vi "Attitude Control Write.vi"(8 "error in (no error)":errorcluster, 9 "Attitude in radians":cluster{"Roll":dbl, "Pitch":dbl, "Yaw":dbl}, 11 "Attitude Control Handle In":T1) -> (0 "error out":errorcluster, 3 "Attitude Control Handle Out":T1)   [LabVIEW 2013, in "lv-attitudecontrol.lvlib"]
uses:
  lv-attitudecontrol.lvlib
  Controls/AttitudeHandle.ctl
  <vilib>/Utility/miscctls.llb/LV3DPointTypeDef.ctl
  <vilib>/picture/3D Picture Control/NI_3D Picture Control.lvlib
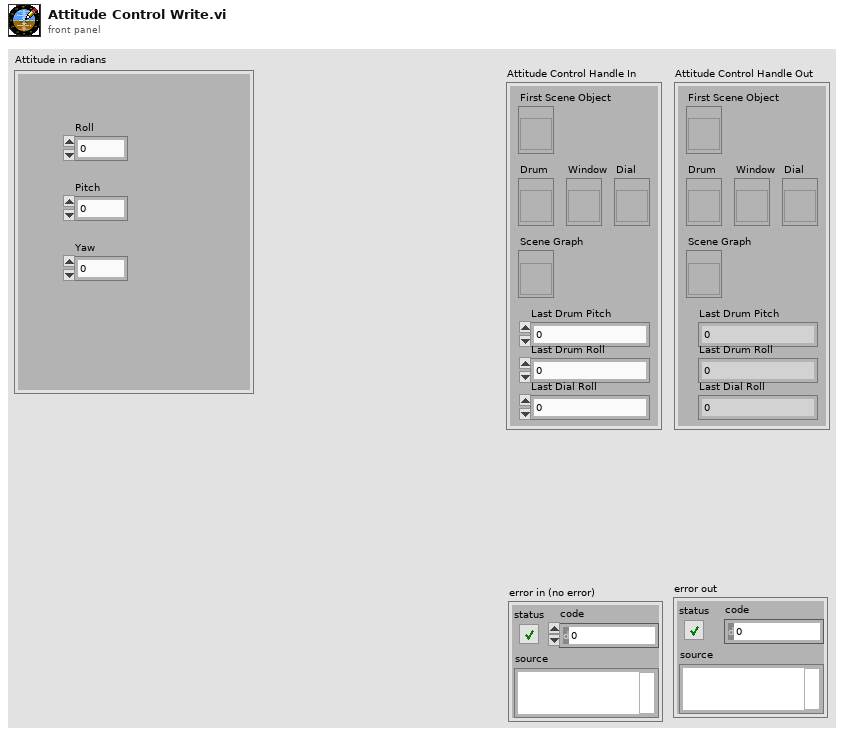
[diagram p1: front panel]
types:
  T1 = typedef "lv-attitudecontrol.lvlib/AttitudeHandle.ctl" = cluster{"First Scene Object":refnum<vi>, "Drum":refnum<vi>, "Window":refnum<vi>, "Dial":refnum<vi>, "Scene Graph":refnum<vi>, "Last Drum Pitch":dbl, "Last Drum Roll ":dbl, "Last Dial Roll":dbl}
  T2 = enum16{"None", "Spherical", "Flying", "Oriented"}
  T3 = typedef "LV3DPointTypeDef.ctl" = cluster{"X":sgl, "Y":sgl, "Z":sgl}
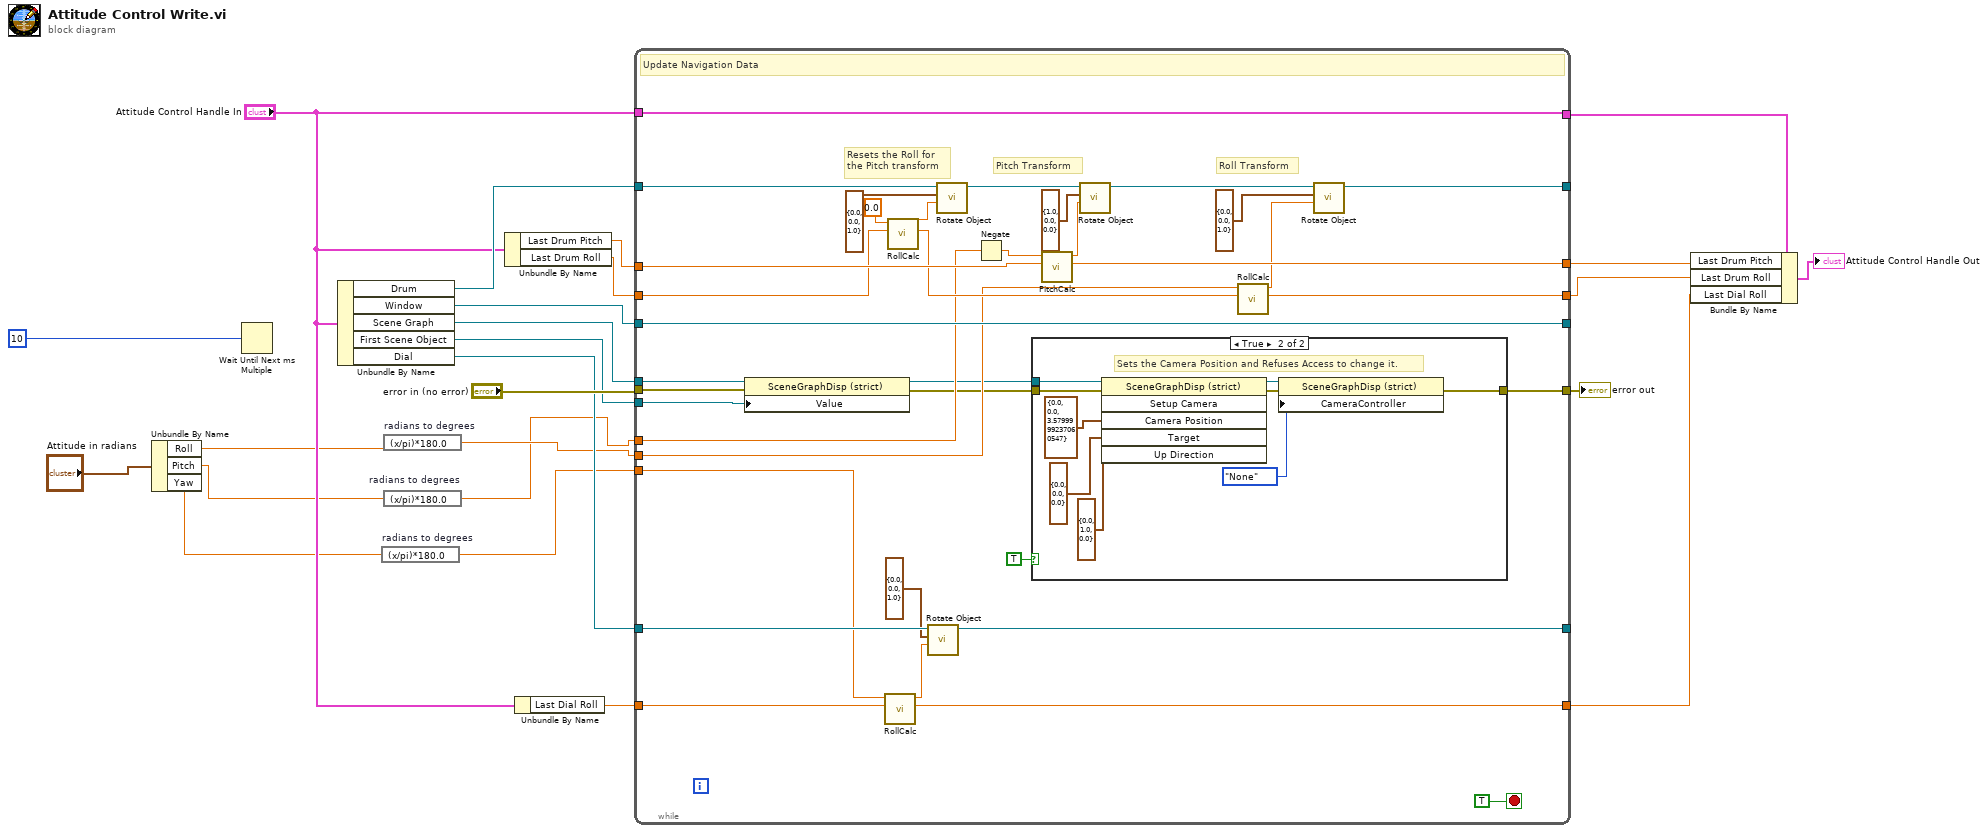
[diagram p0: block diagram]
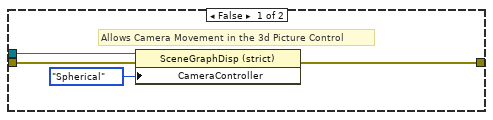
[diagram p2: hidden frame]
diagram:
  n1 = Unbundle By Name("Attitude in radians") -> ("Roll"=w7:dbl, "Pitch"=w6:dbl, "Yaw"=w5:dbl)
  n2 = Wait Until Next ms Multiple(millisecond multiple=u32 10) -> ()  [unwired: 1 out]
  n3 = Unbundle By Name("Attitude Control Handle In") -> ("Drum"=w22:refnum<vi>, "Window"=w23:refnum<vi>, "Scene Graph"=w17:refnum<vi>, "First Scene Object"=w16:refnum<vi>, "Dial"=w15:refnum<vi>)
  n4 = expression code="(x/pi)*180.0" "radians to degrees"(w5) -> (w2:dbl)
  n5 = expression code="(x/pi)*180.0" "radians to degrees"(w7) -> (w3:dbl)
  n6 = expression code="(x/pi)*180.0" "radians to degrees"(w6) -> (w1:dbl)
  n7 = Unbundle By Name("Attitude Control Handle In") -> ("Last Drum Pitch"=w20:dbl, "Last Drum Roll"=w19:dbl)
  n8 = Unbundle By Name("Attitude Control Handle In") -> ("Last Dial Roll"=w18:dbl)
  n9 = while {
    tunnel: w23 -> [w58]
    tunnel: w22 -> [w60]
    tunnel: [w58] -> _
    tunnel: [w57] -> _
    tunnel: w15 -> [w50]
    tunnel: [w48] -> _
    tunnel: "error in (no error)" -> [w31]
    tunnel: [w37] -> w21
    tunnel: w1 -> [w34]
    tunnel: w3 -> [w33]
    tunnel: w2 -> [w32]
    tunnel: w17 -> [w26]
    tunnel: w16 -> [w30]
    tunnel: "Attitude Control Handle In" -> [w25]
    tunnel: [w25] -> w12
    tunnel: w20 -> [w55]
    tunnel: [w54] -> w11
    tunnel: w19 -> [w52]
    tunnel: [w56] -> w10
    tunnel: w18 -> [w51]
    tunnel: [w49] -> w9
    stop <- TRUE stop-if-true
    # "Roll Transform"
    # "Resets the Roll for \nthe Pitch transform"
    # "Pitch Transform"
    # "Update Navigation Data"
    n10 = property on="Property Node" class="SceneGraphDisp (strict)"(reference=w26, error in=w31, "Value"=w30) -> (reference out=w28:refnum<vi>, error out=w29:errorcluster)
    n11 = call "RollCalc.vi"("Previous Roll Value"=w51, "Roll Input"=w32) -> ("New Roll Value"=w49:dbl, "Adjustment to be Made"=w47:dbl)  [unwired: 8 in]
    n12 = call "RollCalc.vi"("Previous Roll Value"=w52, "Roll Input"=sgl 0.0 ("Angle")) -> ("New Roll Value"=w53:dbl, "Adjustment to be Made"=w42:dbl)  [unwired: 8 in]
    n13 = call <vilib>:"Rotate Object.vi"("Angle"=w47, "Axis"=cluster{"X":sgl, "Y":sgl, "Z":sgl} {"X"=0.0, "Y"=0.0, "Z"=1.0} ("Axis 2"), "Scene.Object In"=w50) -> ("Scene.Object Out"=w48:refnum<vi>)  [unwired: 7 in, 1 out]
    n14 = call <vilib>:"Rotate Object.vi"("Angle"=w42, "Axis"=cluster{"X":sgl, "Y":sgl, "Z":sgl} {"X"=0.0, "Y"=0.0, "Z"=1.0} ("Axis 2"), "Scene.Object In"=w60) -> ("Scene.Object Out"=w43:refnum<vi>)  [unwired: 7 in, 1 out]
    n15 = Negate(x=w34) -> (-x=w35:dbl)
    n16 = case shown="True" TRUE {
      tunnel: [w62 w67] -> w37
      tunnel: w29 -> [w64 w69]
      tunnel: w28 -> [w61 w66]
      frame False {
        # "Allows Camera Movement in the 3d Picture Control"
        n17 = property on="Property Node" class="SceneGraphDisp (strict)"(reference=w61, error in=w64, "CameraController"=T2."Spherical" ("Camera Controller:Type")) -> (error out=w62:errorcluster)  [unwired: 1 out]
      }
      frame True {
        # "Sets the Camera Position and Refuses Access to change it."
        n18 = invoke on="Invoke Node" class="SceneGraphDisp (strict)" method="Setup Camera"(reference=w66, error in=w69, "Camera Position"=T3 {"X"=0.0, "Y"=0.0, "Z"=3.58}, "Target"=T3 {"X"=0.0, "Y"=0.0, "Z"=0.0}, "Up Direction"=T3 {"X"=0.0, "Y"=1.0, "Z"=0.0}) -> (reference out=w65:refnum<vi>, error out=w68:errorcluster)  [unwired: 1 in, 4 out]
        n19 = property on="Property Node" class="SceneGraphDisp (strict)"(reference=w65, error in=w68, "CameraController"=T2."None" ("Camera Controller:Type")) -> (error out=w67:errorcluster)  [unwired: 1 out]
      }
    }
    n20 = call "PitchCalc.vi"("Previous Pitch Value"=w55, "Pitch Control"=w35) -> ("New Pitch Value"=w54:dbl, "Adjustment to be made"=w44:dbl)  [unwired: 8 in]
    n21 = call <vilib>:"Rotate Object.vi"("Angle"=w44, "Axis"=cluster{"X":sgl, "Y":sgl, "Z":sgl} {"X"=1.0, "Y"=0.0, "Z"=0.0} ("Axis 2"), "Scene.Object In"=w43) -> ("Scene.Object Out"=w59:refnum<vi>)  [unwired: 7 in, 1 out]
    n22 = call "RollCalc.vi"("Previous Roll Value"=w53, "Roll Input"=w33) -> ("New Roll Value"=w56:dbl, "Adjustment to be Made"=w38:dbl)  [unwired: 8 in]
    n23 = call <vilib>:"Rotate Object.vi"("Angle"=w38, "Axis"=cluster{"X":sgl, "Y":sgl, "Z":sgl} {"X"=0.0, "Y"=0.0, "Z"=1.0} ("Axis 2"), "Scene.Object In"=w59) -> ("Scene.Object Out"=w57:refnum<vi>)  [unwired: 7 in, 1 out]
  }
  "error out" <- w21
  n24 = Bundle By Name(cluster=w12, "Last Drum Pitch"=w11, "Last Drum Roll"=w10, "Last Dial Roll"=w9) -> (→"Attitude Control Handle Out":T1)
